vi "write duty cycle to single relay.vi"(7 "index":i32, 8 "error in (no error)":errorcluster, 9 "Frequency [Hz]":dbl=1.0 format="%#_13g", 10 "Duty Cycle [%]":dbl=10.0 format="%#_13g", 11 "hardware in":refnum<class "hardware.lvclass">) -> (0 "error out":errorcluster, 3 "hardware out":refnum<class "hardware.lvclass">)   [LabVIEW 2025, in "hardware.lvclass"]
uses:
  hardware.lvclass
  hardware.lvclass/hardware.ctl
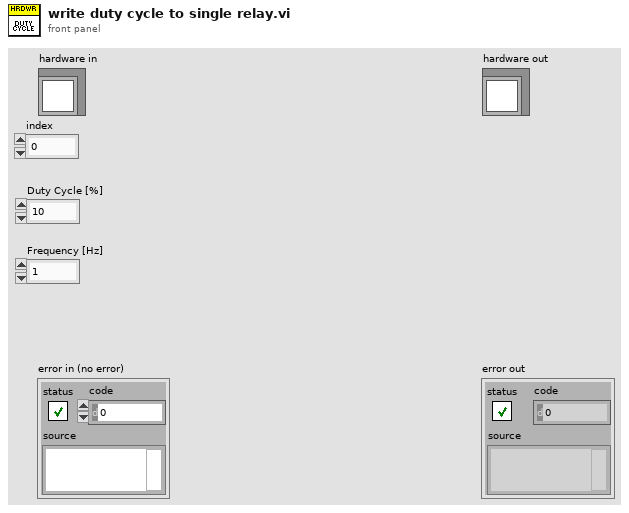
[diagram p1: front panel]
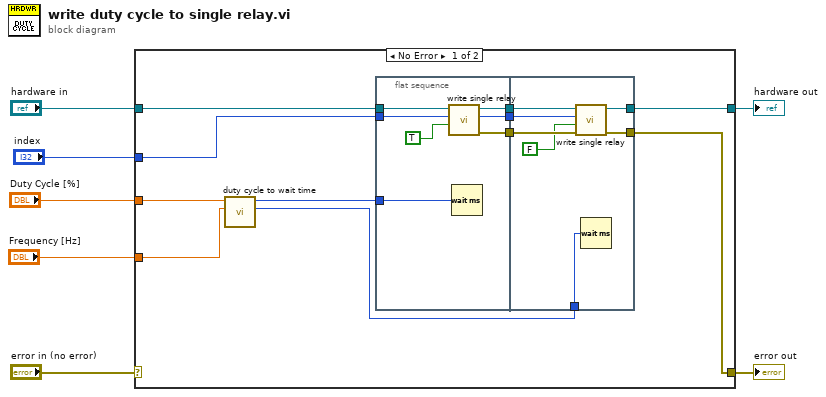
[diagram p0: block diagram]
diagram:
  n1 = case shown="No Error" "error in (no error)" {
    selector: "error in (no error)" -> [_ w33]
    tunnel: [w12 w33] -> w6
    tunnel: [w13 w32] -> w4
    tunnel: "hardware in" -> [w18 w32]
    tunnel: "index" -> [w17 _]
    tunnel: "Duty Cycle [%]" -> [w11 _]
    tunnel: "Frequency [Hz]" -> [w10 _]
    frame No Error {
      n2 = call "duty cycle to wait time.vi"("Frequency [Hz]"=w10, "Duty Cycle [%]"=w11) -> ("Off Time [ms]"=w8:u32, "On Time [ms]"=w9:u32)  [unwired: 8 in]
      n3 = flat-sequence {
        tunnel: w18 -> [w24]
        tunnel: w17 -> [w20]
        tunnel: [w22] -> w16
        tunnel: [w21] -> w15
        tunnel: [w20] -> w14
        tunnel: w9 -> [w19]
        tunnel: w16 -> [w31]
        tunnel: w15 -> [w30]
        tunnel: w14 -> [w29]
        tunnel: [w27] -> w13
        tunnel: [w26] -> w12
        tunnel: w8 -> [w25]
        frame #0 {
          n4 = call-dynamic "write single relay.vi"("on/off"=TRUE, "index"=w20, "hardware in"=w24) -> ("error out"=w21:errorcluster, "hardware out"=w22:refnum<class "hardware.lvclass">)  [unwired: 7 in]
          n5 = Wait (ms)(milliseconds to wait=w19) -> ()  [unwired: 1 out]
        }
        frame #1 {
          n6 = call-dynamic "write single relay.vi"("error in (no error)"=w30, "on/off"=FALSE, "index"=w29, "hardware in"=w31) -> ("error out"=w26:errorcluster, "hardware out"=w27:refnum<class "hardware.lvclass">)  [unwired: 6 in]
          n7 = Wait (ms)(milliseconds to wait=w25) -> ()  [unwired: 1 out]
        }
      }
    }
    frame Error {
    }
  }
  "error out" <- w6
  "hardware out" <- w4
